vi "Manual Override Manipulator Controls.vi"(9 "Manual Override Scaling":dbl, 10 "Deadband":dbl, 11 "Operator Axes":dbl[](array[numeric])) -> (2 "Manul Override Requested?":bool, 3 "Manual Override Data":cluster{"Wrist Power":dbl, "Cascade Power":dbl})   [LabVIEW 2020]
uses:
  <vilib>/Rock Robotics/WPI/Joystick/XBox Axes Indexer.ctl
  e6c857f1-48c5-43ef-8972-3c5f5400eeaf.vi
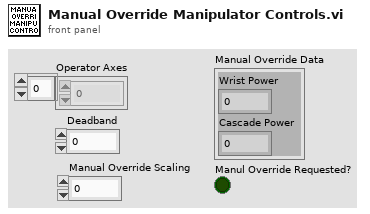
[diagram p1: front panel]
types:
  T1 = typedef "XBox Axes Indexer.ctl" = enum16{"Left X", "Left Y", "Left Trigger", "Right Trigger", "Right X", "Right Y"}
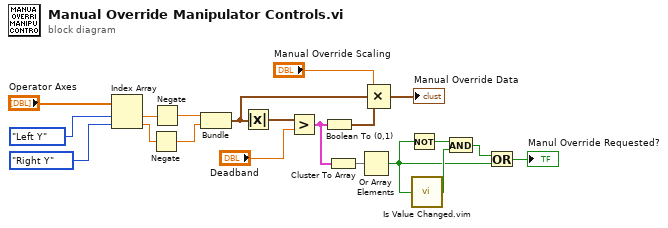
[diagram p0: block diagram]
diagram:
  n1 = Index Array(array="Operator Axes", index #1=XBox_Axes_Indexer."Left Y" ("XBox Axes"), index #2=XBox_Axes_Indexer."Right Y" ("XBox Axes")) -> (element #1=w17:dbl, element #2=w16:dbl)
  n2 = Negate(x=w16) -> (-x=w14:dbl)
  n3 = Negate(x=w17) -> (-x=w15:dbl)
  n4 = Bundle(w15, w14) -> (w11:cluster{dbl, dbl})  [unwired: 1 in]
  n5 = Absolute Value(x=w11) -> (abs(x)=w13:cluster{dbl, dbl})
  n6 = Greater?(x=w13, y="Deadband") -> (0:w7:cluster{bool, bool})
  n7 = Boolean To (0,1)(Boolean=w7) -> (0, 1=w8:cluster{i16, i16})
  n8 = Cluster To Array(cluster=w7) -> (array=w6:bool[])
  n9 = Or Array Elements(Boolean array=w6) -> (logical OR=w2:bool)
  n10 = Compound Arithmetic op=MULTIPLY("Manual Override Scaling", w11, w8) -> (→"Manual Override Data":cluster{dbl, dbl})
  n11 = Not(x=w2) -> (.not. x?=w5:bool)
  n12 = call "Is Value Changed.vim"("value"=w2) -> ("changed or first call?"=w4:bool)
  n13 = And(x=w5, y=w4) -> (x .and. y?=w3:bool)
  n14 = Or(x=w3, y=w2) -> (x .or. y?=→"Manul Override Requested?":bool)
